vi "Save-image-with-right-filetype.vi"(6 "Image file type":enum16{"JPG", "BMP", "PNG"}(ring), 7 "Color Palette":cluster{"Red":u8, "Green":u8, "Blue":u8}[](array[cluster]), 8 "error in":errorcluster, 9 "Filename":string, 10 "Filepath and name":path, 11 "Image in":T1) -> (0 "error IO":errorcluster)   [LabVIEW 2013, in "CameraVision.lvlib" / "CV-Storage.lvclass"]
uses:
  CV-Storage.lvclass
  <vilib>/vision/Image Controls.llb/IMAQ Image.ctl
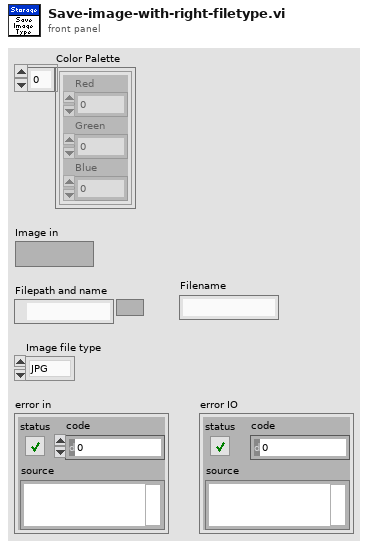
[diagram p1: front panel]
types:
  T1 = typedef "IMAQ Image.ctl" = refnum<image>
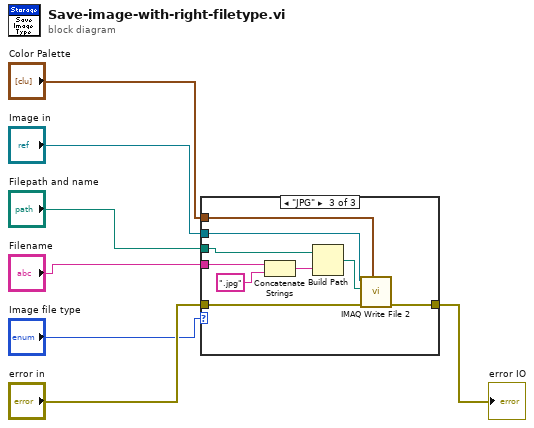
[diagram p0: block diagram]
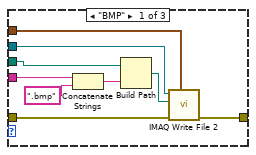
[diagram p2: hidden frame]
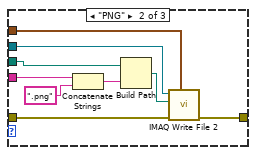
[diagram p3: hidden frame]
diagram:
  n1 = case shown="\"JPG\"" "Image file type" {
    tunnel: "Image in" -> [w16 w25 w34]
    tunnel: "Filepath and name" -> [w11 w19 w30]
    tunnel: "error in" -> [w15 w24 w33]
    tunnel: [w14 w23 w32] -> w5
    tunnel: "Color Palette" -> [w13 w22 w31]
    tunnel: "Filename" -> [w8 w17 w26]
    frame "BMP" {
      n2 = Concatenate Strings(w8, ".bmp" ("name or relative path")) -> (w9:string)
      n3 = Build Path(base path=w11, name or relative path=w9) -> (appended path=w10:path)
      n4 = call-poly "IMAQ Write File 2"("Color Palette"=w13, "error in (no error)"=w15, "File Path"=w10, "Image"=w16) -> ("error out"=w14:errorcluster)  [unwired: 6 in, 1 out]
    }
    frame "PNG" {
      n5 = Concatenate Strings(w17, ".png" ("name or relative path")) -> (w18:string)
      n6 = Build Path(base path=w19, name or relative path=w18) -> (appended path=w20:path)
      n7 = call-poly "IMAQ Write File 2"("Color Palette"=w22, "error in (no error)"=w24, "File Path"=w20, "Image"=w25) -> ("error out"=w23:errorcluster)  [unwired: 6 in, 1 out]
    }
    frame "JPG" {
      n8 = Concatenate Strings(w26, ".jpg" ("name or relative path")) -> (w27:string)
      n9 = Build Path(base path=w30, name or relative path=w27) -> (appended path=w29:path)
      n10 = call-poly "IMAQ Write File 2"("Color Palette"=w31, "error in (no error)"=w33, "File Path"=w29, "Image"=w34) -> ("error out"=w32:errorcluster)  [unwired: 6 in, 1 out]
    }
  }
  "error IO" <- w5
